vi "Trigger Tester Connection.vi"(8 "error in":errorcluster, 11 "ECU Read Data":T1[](array[typedef]) {"ID" format="%01x"; "Payload" format="%02x"}) -> (0 "error out":errorcluster)   [LabVIEW 2024, in "RT Management.lvlib"]
uses:
  RT Management.lvlib
  Shared Modules/CAN Commands Interpreter/CAN Frame Data.ctl
  ECU Internal Communications/Notifiers - Get.vi
  ECU Internal Communications/ECU InterComm.lvlib
  Shared Modules/CAN Commands Interpreter/CAN Commands.lvlib
panel:
  out "Tester Connected":bool
  out "Tester Found":bool
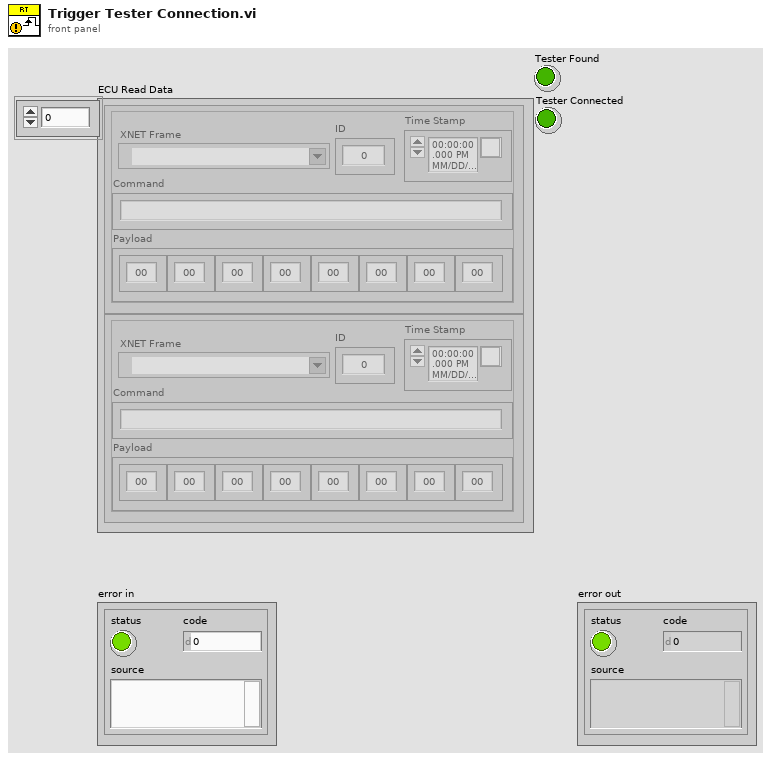
[diagram p1: front panel]
types:
  T1 = typedef "CAN Commands.lvlib/CAN Frame Data.ctl" = cluster{"Command":string, "XNET Frame":refnum<k21>, "Payload":u8[], "ID":u32, "Time Stamp":timestamp}
  T2 = typedef "ECU InterComm.lvlib/ECU Notifiers.ctl" = cluster{"Tester Detected":refnum<notifier>, "STOP Reading":refnum<notifier>}
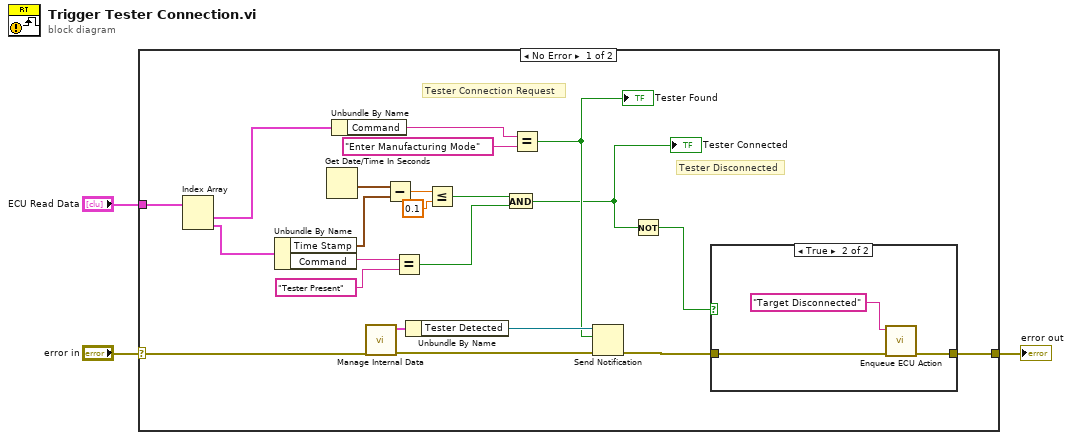
[diagram p0: block diagram]
diagram:
  n1 = case shown="No Error" "error in" {
    selector: "error in" -> [w25 w30]
    tunnel: [w5 w30] -> w3
    tunnel: "ECU Read Data" -> [w24 _]
    frame No Error {
      # "Tester Disconnected"
      # "Tester Connection Request"
      n2 = Index Array(array=w24) -> (element #1=w21:T1, element #2=w13:T1)  [unwired: 2 in]
      n3 = Unbundle By Name(w13) -> ("Time Stamp"=w15:timestamp, "Command"=w19:string)
      n4 = Get Date/Time In Seconds() -> (seconds since 1Jan1904=w14:timestamp)
      n5 = Unbundle By Name(w21) -> ("Command"=w22:string)
      n6 = call-poly "Manage Internal Data.vi"("error in"=w25) -> ("error out"=w11:errorcluster, "ECU Notifiers"=w7:T2)  [unwired: 9 in]
      n7 = Subtract(x=w14, y=w15) -> (x-y=w16:dbl)
      n8 = Equal?(x=w19, y="Tester Present") -> (x = y?=w20:bool)
      n9 = Unbundle By Name(w7) -> ("Tester Detected"=w10:refnum<notifier>)
      n10 = Less Or Equal?(x=w16, y=0.1) -> (x <= y?=w18:bool)
      n11 = And(x=w18, y=w20) -> (x .and. y?=w8:bool)
      "Tester Connected" <- w8
      n12 = Equal?(x=w22, y="Enter Manufacturing Mode") -> (x = y?=w9:bool)
      "Tester Found" <- w9
      n13 = Send Notification(notification=w9, notifier=w10, error in (no error)=w11) -> (error out=w6:errorcluster)  [unwired: 1 out]
      n14 = Not(x=w8) -> (.not. x?=w4:bool)
      n15 = case shown="True" w4 {
        tunnel: w6 -> [w26 w29]
        tunnel: [w26 w28] -> w5
        frame False {
        }
        frame True {
          n16 = call "Enqueue ECU Action.vi"("error in"=w29, "Message"="Target Disconnected") -> ("error out"=w28:errorcluster)  [unwired: 9 in]
        }
      }
    }
    frame Error {
    }
  }
  "error out" <- w3
